vi "Forward Remote Events.vi"(7 "Node":string, 8 "error in (no error)":errorcluster, 10 "Data":T1, 11 "Event Reporter Module in":refnum<class "Event Reporter Module.lvclass">) -> (0 "error out":errorcluster, 3 "Event Reporter Module out":refnum<class "Event Reporter Module.lvclass">)   [LabVIEW 2020, in "Volatus.lvlib" / "Event Reporter Module.lvclass"]
uses:
  Event Reporter Module.lvclass
  messages/Events/Data.ctl
  messages/Event/Data.ctl
  messages/EventLevel/Enumeration.ctl
  messages/Error/Data.ctl
  Event Reporter Module.lvclass/Event Reporter Module.ctl
  Event.ctl
  Event Level.ctl
  MessageQ/MessageQ.lvclass/MessageQ.ctl
  MessageQ/MessageQ.lvclass
  lv-vecto/Vecto/Vecto.lvlib
  Volatus.lvlib
  messages/Error/Error.lvlib
  messages/EventLevel/EventLevel.lvlib
  messages/Event/Event.lvlib
  messages/Events/Events.lvlib
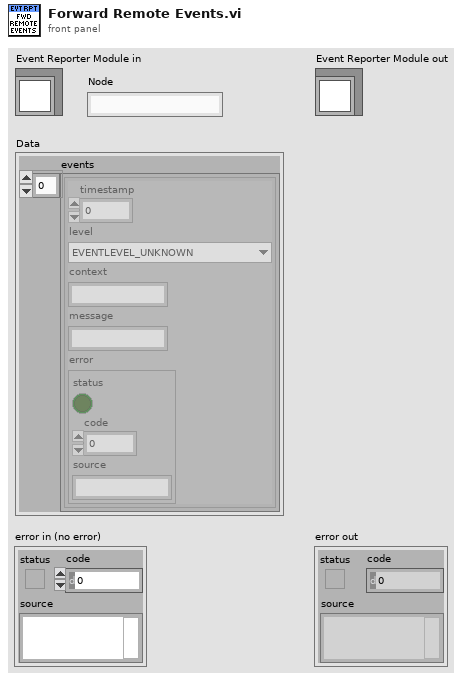
[diagram p1: front panel]
types:
  T1 = typedef "Events.lvlib/Data.ctl" = cluster{"events":T2[]}
  T2 = typedef "Event.lvlib/Data.ctl" = cluster{"timestamp":i64, "level":T3, "context":string, "message":string, "error":T4}
  T3 = typedef "EventLevel.lvlib/Enumeration.ctl" = enum16{"EVENTLEVEL_UNKNOWN", "EVENTLEVEL_DEBUG", "EVENTLEVEL_INFO", "EVENTLEVEL_WARNING", "EVENTLEVEL_ERROR"}
  T4 = typedef "Error.lvlib/Data.ctl" = errorcluster
  T5 = typedef "Volatus.lvlib/Event.ctl" = cluster{"Time Stamp":timestamp, "Event Level":T6, "Context":string, "Message":string, "Error":errorcluster, "Node":string}
  T6 = typedef "Volatus.lvlib/Event Level.ctl" = enum16{"Debug", "Info", "Warning", "Error"}
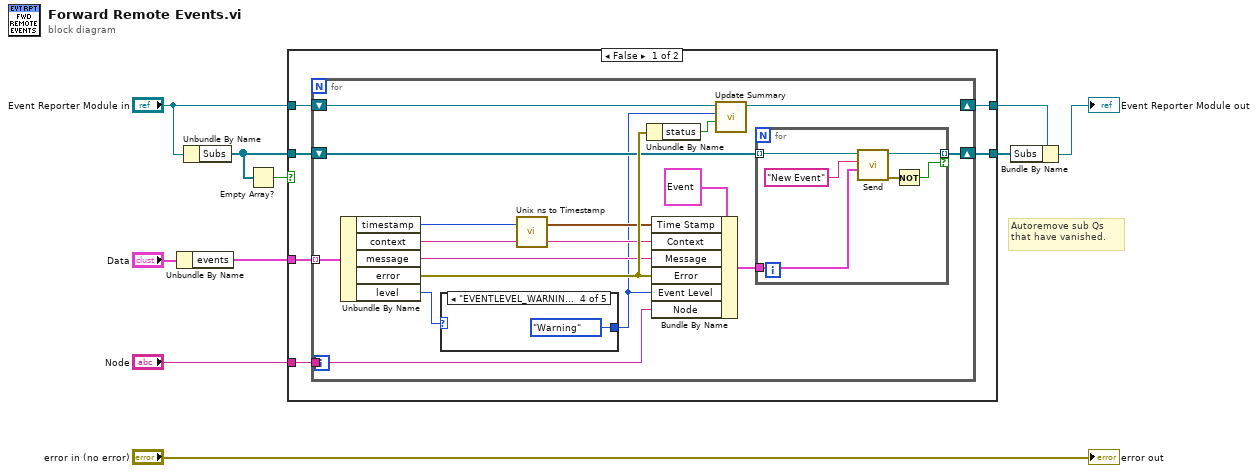
[diagram p0: block diagram]
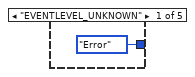
[diagram p2: hidden frame]
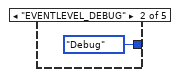
[diagram p3: hidden frame]
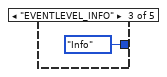
[diagram p4: hidden frame]
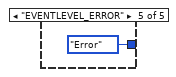
[diagram p5: hidden frame]
diagram:
  # "Autoremove sub Qs that have vanished."
  n1 = Unbundle By Name("Data") -> ("events"=w8:T2[])
  n2 = Unbundle By Name("Event Reporter Module in") -> ("Subs"=w6:refnum<class "MessageQ.lvclass">[])
  n3 = Empty Array?(array=w6) -> (empty?=w5:bool)
  n4 = case shown="False" w5 {
    tunnel: w8 -> [w16 _]
    tunnel: "Node" -> [w15 _]
    tunnel: w6 -> [w14 w45]
    tunnel: [w13 w45] -> w3
    tunnel: "Event Reporter Module in" -> [w12 w44]
    tunnel: [w11 w44] -> w1
    frame False {
      n5 = for {
        tunnel: w16 -> [w31] mode=indexing
        tunnel: w15 -> [w26]
        shift-right: [w21] -> w13
        shift-left: w14 -> [w30]
        shift-right: [w17] -> w11
        shift-left: w12 -> [w20]
        n6 = Unbundle By Name(w31) -> ("timestamp"=w29:i64, "context"=w24:string, "message"=w25:string, "error"=w32:T4, "level"=w23:T3)
        n7 = case shown="\"EVENTLEVEL_WARNING\"" w23 {
          tunnel: [Event_Level."Error" ("Event Level") Event_Level."Debug" ("Event Level") Event_Level."Info" ("Event Level") Event_Level."Warning" ("Event Level") Event_Level."Error" ("Event Level")] -> w19
          frame "EVENTLEVEL_UNKNOWN" {
          }
          frame "EVENTLEVEL_DEBUG" {
          }
          frame "EVENTLEVEL_INFO" {
          }
          frame "EVENTLEVEL_WARNING" {
          }
          frame "EVENTLEVEL_ERROR" {
          }
        }
        n8 = call "Unix ns to Timestamp.vi"("Unix ns"=w29) -> ("Time Stamp"=w27:timestamp)  [unwired: 2 in]
        n9 = Unbundle By Name(w32) -> ("status"=w18:bool)
        n10 = Bundle By Name(cluster=T5 {"Time Stamp"=timestamp(0 s since 1904-01-01), "Event Level"=enum."Info", "Context"="", "Message"="", "Error"={"status"=FALSE, "code"=0, "source"=""}, "Node"=""} ("Event"), "Time Stamp"=w27, "Context"=w24, "Message"=w25, "Error"=w32, "Event Level"=w19, "Node"=w26) -> (w22:T5)
        n11 = call "Update Summary.vi"("Error Status"=w18, "Level"=w19, "Event Reporter Module in"=w20) -> ("Event Reporter Module out"=w17:refnum<class "Event Reporter Module.lvclass">)  [unwired: 7 in, 1 out]
        n12 = for {
          tunnel: w30 -> [w43] mode=indexing
          tunnel: w22 -> [w41]
          tunnel: [w40] -> w21 mode=indexing if=w38
          n13 = call "Send.vi"("Data"=w41, "ID"="New Event", "MessageQ in"=w43) -> ("error out"=w39:errorcluster, "MessageQ out"=w40:refnum<class "MessageQ.lvclass">)  [unwired: 7 in]
          n14 = Not(x=w39) -> (.not. x?=w38:bool)
        }
      }
    }
    frame True {
    }
  }
  n15 = Bundle By Name(cluster=w1, "Subs"=w3) -> (→"Event Reporter Module out":refnum<class "Event Reporter Module.lvclass">)
  "error out" <- "error in (no error)"
